vi "Facade.vi"(0 "Data In":T4, 2 "Display State In":T2={"State 1"={"BG"=0, "FG"=0}, "State 0"={"BG"=0, "FG"=0}, "State 2"={"BG"=0, "FG"=0}, "State 3"={"BG"=0, "FG"=0}, "Shortcut Menu"=enum."Do left-click popup"}, 3 "Container State":T3) -> (6 "Data Out":T4, 7 "Display State Out":T2={"State 1"={"BG"=0, "FG"=0}, "State 0"={"BG"=0, "FG"=0}, "State 2"={"BG"=0, "FG"=0}, "State 3"={"BG"=0, "FG"=0}, "Shortcut Menu"=enum."Do left-click popup"}, 8 "Action":T1)   [LabVIEW 2011, in "Led.xctl"]
uses:
  Led.xctl
  TD_Status.ctl
  <vilib>/_xctls/Container State.ctl
  State.ctl
  <vilib>/_xctls/Action.ctl
  <vilib>/_xctls/XControlSupport.lvlib
panel:
  # "How to resize the XCTL to 20x20...\n\n1. Open the Facade.vi windows run-time position properties\n2. Select the Position, custom... set the panel size to 20x20.\n3. Save and close de Facade.vi\n4. Open the GUI_Led.vi, drag the XCTL into the FrontPanel\n5. Open the Facade.vi (the vi will be automatically size to 20x20 because it was call in runtime\n6. Close the Gui_Led.vi (no need to save)\n7. Facade.vi not become in edit mode with the 20x20 size, so save it like that with CTRL+S\n8. Close Facade.vi\n9. Enjoy your XCTL of 20x20 size!!!"
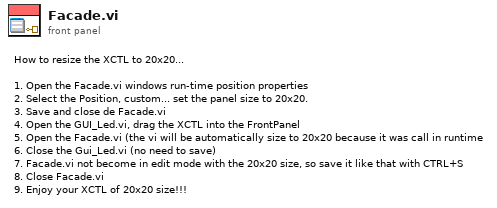
[diagram p1: front panel]
types:
  T1 = typedef "XControlSupport.lvlib/Action.ctl" = cluster{"Data Changed?":bool, "State Changed?":bool, "Action Name":string}
  T2 = typedef "Led.xctl/State.ctl" = cluster{"State 1":cluster{"BG":u32, "FG":u32}, "State 0":cluster{"BG":u32, "FG":u32}, "State 2":cluster{"BG":u32, "FG":u32}, "State 3":cluster{"BG":u32, "FG":u32}, "Shortcut Menu":enum16{"Treat normally", "Do left-click popup"}}
  T3 = typedef "XControlSupport.lvlib/Container State.ctl" = cluster{"Indicator?":bool, "Run Mode?":bool, " Refnum":refnum<vi>}
  T4 = typedef "Led.xctl/TD_Status.ctl" = enum16{"Disconnected", "Connected", "Connecting", "Error"}
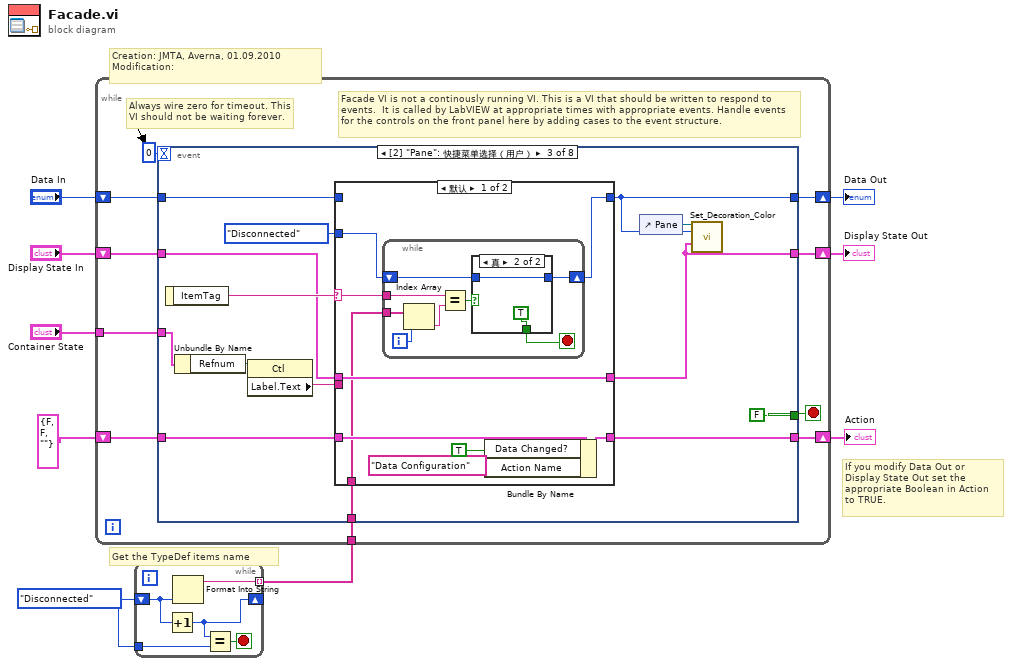
[diagram p0: block diagram]
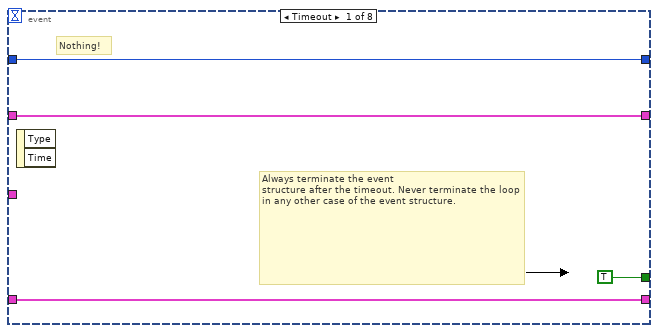
[diagram p2: hidden frame]
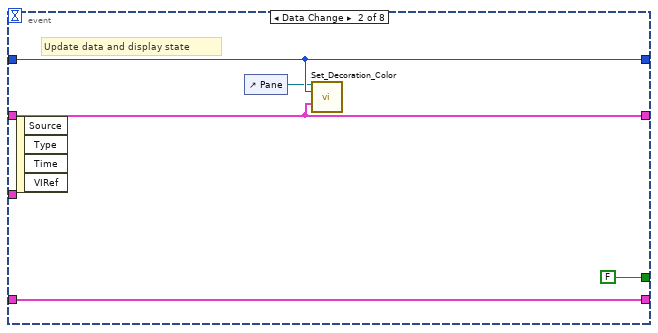
[diagram p3: hidden frame]
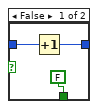
[diagram p4: hidden frame]
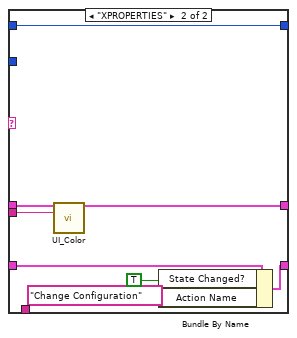
[diagram p5: hidden frame]
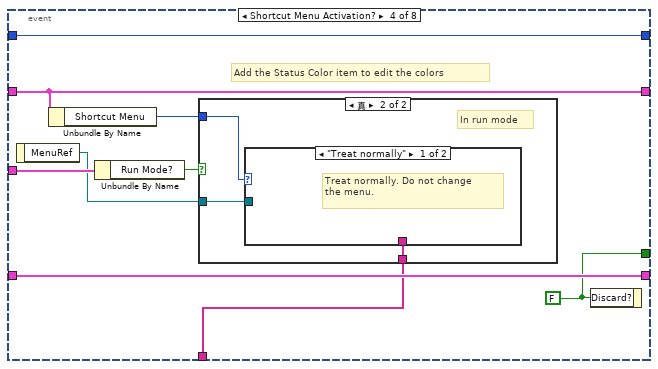
[diagram p6: hidden frame]
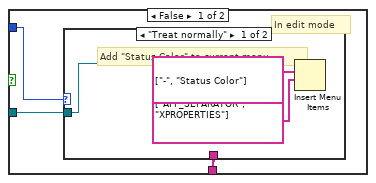
[diagram p7: hidden frame]
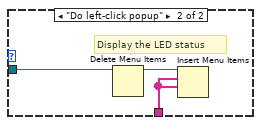
[diagram p8: hidden frame]
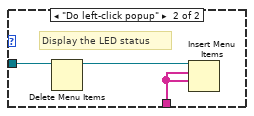
[diagram p9: hidden frame]
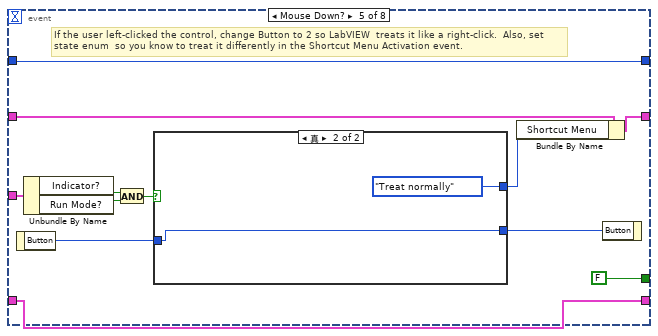
[diagram p10: hidden frame]
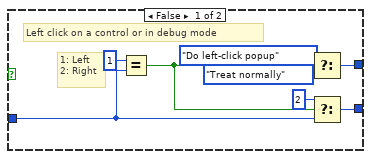
[diagram p11: hidden frame]
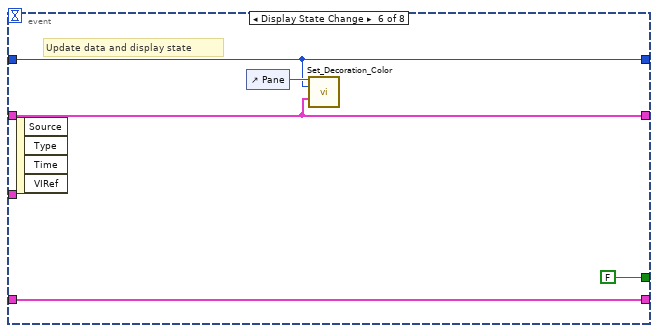
[diagram p12: hidden frame]
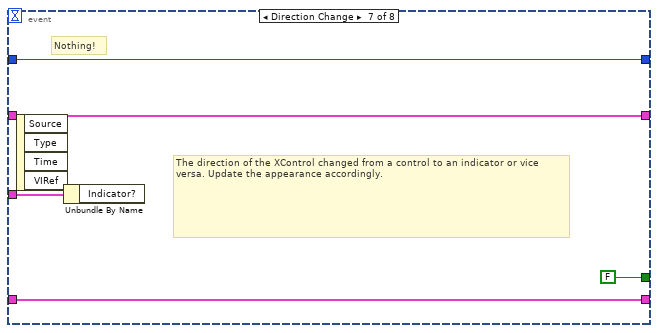
[diagram p13: hidden frame]
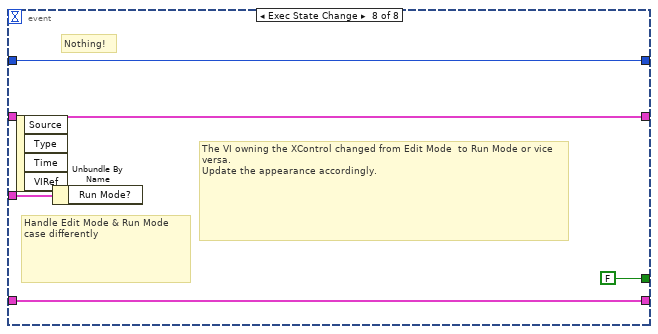
[diagram p14: hidden frame]
diagram:
  w1 = TD_Status."Disconnected" ("Status")
  # "Get the TypeDef items name"
  # "Creation: JMTA, Averna, 01.09.2010 \nModification:"
  # "If you modify Data Out or\nDisplay State Out set the\nappropriate Boolean in Action\nto TRUE."
  n1 = while {
    shift-right: [w11] -> _
    shift-left: w1 -> [w13]
    tunnel: [w12] -> w2 mode=indexing
    tunnel: w1 -> [w10]
    stop <- w14 stop-if-true
    n2 = Increment(x=w13) -> (x+1=w11:T4)
    n3 = Format Into String(w13) -> (resulting string=w12:string)  [unwired: 3 in, 1 out]
    n4 = Equal?(x=w11, y=w10) -> (x = y?=w14:bool)
  }
  n5 = while {
    shift-right: [w23] -> w6
    shift-left: "Display State In" -> [w24]
    tunnel: "Container State" -> [w20]
    shift-right: [w18] -> w9
    shift-left: "Data In" -> [w19]
    shift-right: [w16] -> w4
    shift-left: T1 {"Data Changed?"=FALSE, "State Changed?"=FALSE, "Action Name"=""} ("Action") -> [w17]
    tunnel: w2 -> [w15]
    stop <- w22 stop-if-true
    # "Facade VI is not a continously running VI. This is a VI that should be written to respond to events.  It is called by LabVIEW at appropriate times with appropriate events. Handle events for the controls on the front panel here by adding cases to the event structure."
    # "Always wire zero for timeout. This\nVI should not be waiting forever."
    n6 = event shown="[2] \"Pane\": 快捷菜单选择（用户）" {
      selector: _ -> [_ _ _ _ _ _ _ _]
      dyn-events: _ -> [_ _ _ _ _ _ _ _]
      timeout: 0 -> [_ _ _ _ _ _ _ _]
      tunnel: w24 -> [w26 w30 w35 w81 w107 w125 w132 w137]
      tunnel: [w26 w30 w38 w81 w108 w125 w132 w137] -> w23
      tunnel: [TRUE FALSE ("Discard?") FALSE ("Discard?") w83 FALSE ("Discard?") FALSE ("Discard?") FALSE ("Discard?") FALSE ("Discard?")] -> w22
      tunnel: w20 -> [_ _ w47 w86 w105 _ w133 w138]
      tunnel: w19 -> [w25 w31 w42 w85 w111 w124 w131 w136]
      tunnel: [w25 w31 w37 w85 w111 w124 w131 w136] -> w18
      tunnel: [w27 w33 w41 w84 w110 w128 w130 w135] -> w16
      tunnel: w17 -> [w27 w33 w40 w84 w110 w128 w130 w135]
      tunnel: w15 -> [_ _ w36 w79 _ _ _ _]
      event Timeout {
        # "Nothing!"
        # "Always terminate the event\nstructure after the timeout. Never terminate the loop in any other case of the event structure."
        n7 = event-data() -> ()  [unwired: 1 in, 2 out]
      }
      event Data Change {
        # "Update data and display state"
        n8 = event-data() -> ()  [unwired: 1 in, 4 out]
        n9 = control-ref of="Pane"() -> (w29:refnum<vi>)
        n10 = call "Set_Decoration_Color.vi"("Pane ref"=w29, "Data In"=w31, "Display State In"=w30) -> ()  [unwired: 13 in]
      }
      event Shortcut Menu Selection (User) {
        n11 = event-data() -> ("ItemTag"=w43:string)  [unwired: 1 in]
        n12 = Unbundle By Name(w47) -> ("Refnum"=w46:refnum<vi>)
        n13 = property class="Ctl"(reference=w46) -> ("Label.Text"=w45:string)  [unwired: 1 in, 2 out]
        n14 = case shown="默认" w43 {
          selector: w43 -> [w50 _]
          tunnel: w35 -> [w56 w77]
          tunnel: [w56 w75] -> w38
          tunnel: w45 -> [_ w76]
          tunnel: w42 -> [_ w74]
          tunnel: [w48 w74] -> w37
          tunnel: [w53 w71] -> w41
          tunnel: w40 -> [w52 w70]
          tunnel: w36 -> [w51 _]
          tunnel: TD_Status."Disconnected" ("Status") -> [w49 _]
          frame Default {
            n15 = while {
              tunnel: w51 -> [w63]
              tunnel: w50 -> [w61]
              shift-right: [w58] -> w48
              shift-left: w49 -> [w59]
              i -> [w64]
              stop <- w57 stop-if-true
              n16 = Index Array(array=w63, index=w64) -> (element=w62:string)
              n17 = Equal?(x=w61, y=w62) -> (x = y?=w60:bool)
              n18 = case shown="真" w60 {
                tunnel: w59 -> [w67 w69]
                tunnel: [w66 w69] -> w58
                tunnel: [FALSE TRUE] -> w57
                frame False {
                  n19 = Increment(x=w67) -> (x+1=w66:T4)
                }
                frame True {
                }
              }
            }
            n20 = Bundle By Name(cluster=w52, "Data Changed?"=TRUE, "Action Name"="Data Configuration") -> (w53:T1)
          }
          frame "XPROPERTIES" {
            n21 = call "UI_Color.vi"("State in"=w77, "FP.Title"=w76) -> ("State out"=w75:T2)  [unwired: 12 in, 1 out]
            n22 = Bundle By Name(cluster=w70, "State Changed?"=TRUE ("Data Changed?"), "Action Name"="Change Configuration") -> (w71:T1)
          }
        }
        n23 = control-ref of="Pane"() -> (w39:refnum<vi>)
        n24 = call "Set_Decoration_Color.vi"("Pane ref"=w39, "Data In"=w37, "Display State In"=w38) -> ()  [unwired: 13 in]
      }
      event Shortcut Menu Activation? {
        w83 = FALSE ("Discard?")
        # "Add the Status Color item to edit the colors"
        n25 = event-data() -> ("MenuRef"=w80:refnum<k9>)  [unwired: 1 in]
        n26 = Unbundle By Name(w81) -> ("Shortcut Menu"=w78:enum16{"Treat normally", "Do left-click popup"})
        n27 = Unbundle By Name(w86) -> ("Run Mode?"=w82:bool)
        n28 = case shown="真" w82 {
          tunnel: w78 -> [w89 w98]
          tunnel: w80 -> [w87 w97]
          tunnel: w79 -> [w88 w96]
          frame False {
            # "In edit mode"
            n29 = case shown="\"Treat normally\"" w89 {
              tunnel: w88 -> [_ w94]
              tunnel: w87 -> [w90 w93]
              frame "Treat normally" {
                # "Add \"Status Color\" to current menu"
                n30 = Insert Menu Items(7:string[] ["APP_SEPARATOR", "XPROPERTIES"] ("item names"), 8:string[] ["-", "Status Color"] ("item names"), 9:w90) -> ()  [unwired: 3 in, 3 out]
              }
              frame "Do left-click popup" {
                # "Display the LED status"
                n31 = Delete Menu Items(9:w93) -> (3:w95:refnum<k9>)  [unwired: 3 in, 1 out]
                n32 = Insert Menu Items(7:w94, 8:w94, 9:w95) -> ()  [unwired: 3 in, 3 out]
              }
            }
          }
          frame True {
            # "In run mode"
            n33 = case shown="\"Treat normally\"" w98 {
              tunnel: w97 -> [_ w100]
              tunnel: w96 -> [_ w99]
              frame "Treat normally" {
                # "Treat normally. Do not change\nthe menu."
              }
              frame "Do left-click popup" {
                # "Display the LED status"
                n34 = Delete Menu Items(9:w100) -> (3:w101:refnum<k9>)  [unwired: 3 in, 1 out]
                n35 = Insert Menu Items(7:w99, 8:w99, 9:w101) -> ()  [unwired: 3 in, 3 out]
              }
            }
          }
        }
        n36 = event-data("Discard?"=w83) -> ()  [unwired: 1 in, 1 out]
      }
      event Mouse Down? {
        # "If the user left-clicked the control, change Button to 2 so LabVIEW  treats it like a right-click.  Also, set state enum  so you know to treat it differently in the Shortcut Menu Activation event."
        n37 = event-data() -> ("Button"=w113:u16)  [unwired: 1 in]
        n38 = Unbundle By Name(w105) -> ("Indicator?"=w103:bool, "Run Mode?"=w102:bool)
        n39 = And(x=w103, y=w102) -> (x .and. y?=w104:bool)
        n40 = case shown="真" w104 {
          tunnel: w113 -> [w116 w123]
          tunnel: [w115 w123] -> w112
          tunnel: [w114 enum16{"Treat normally", "Do left-click popup"}."Treat normally" ("Enum")] -> w106
          frame False {
            # "Left click on a control or in debug mode"
            # "1: Left\n2: Right"
            n41 = Equal?(x=u16 1, y=w116) -> (x = y?=w120:bool)
            n42 = Select(t=enum16{"Treat normally", "Do left-click popup"}."Do left-click popup" ("f"), s=w120, f=enum16{"Treat normally", "Do left-click popup"}."Treat normally" ("Enum")) -> (s? t:f=w114:enum16{"Treat normally", "Do left-click popup"})
            n43 = Select(t=u16 2, s=w120, f=w116) -> (s? t:f=w115:u16)
          }
          frame True {
          }
        }
        n44 = Bundle By Name(cluster=w107, "Shortcut Menu"=w106) -> (w108:T2)
        n45 = event-data("Button"=w112) -> ()  [unwired: 1 in, 1 out]
      }
      event Display State Change {
        # "Update data and display state"
        n46 = event-data() -> ()  [unwired: 1 in, 4 out]
        n47 = control-ref of="Pane"() -> (w126:refnum<vi>)
        n48 = call "Set_Decoration_Color.vi"("Pane ref"=w126, "Data In"=w124, "Display State In"=w125) -> ()  [unwired: 13 in]
      }
      event Direction Change {
        # "Nothing!"
        # "The direction of the XControl changed from a control to an indicator or vice versa. Update the appearance accordingly."
        n49 = event-data() -> ()  [unwired: 1 in, 4 out]
        n50 = Unbundle By Name(w133) -> ()  [unwired: 1 out]
      }
      event Exec State Change {
        # "Nothing!"
        # "The VI owning the XControl changed from Edit Mode  to Run Mode or vice versa.\nUpdate the appearance accordingly."
        # "Handle Edit Mode & Run Mode\ncase differently"
        n51 = event-data() -> ()  [unwired: 1 in, 4 out]
        n52 = Unbundle By Name(w138) -> ()  [unwired: 1 out]
      }
    }
  }
  "Display State Out" <- w6
  "Data Out" <- w9
  "Action" <- w4
